vi "Dpc Get First Error.vi"(8 "error in (no error)":errorcluster, 11 "hif":u32) -> (0 "error out":errorcluster, 2 "function return":i32, 3 "hif out":u32)   [LabVIEW 2011, in "LVH-Adept.lvlib" / "DPCUTIL.lvlib"]
doc: "DPCAPI ERC DpcGetFirstError(HANDLE hif);"
uses:
  DPCUTIL.lvlib
  Resources/dpcutil.dll
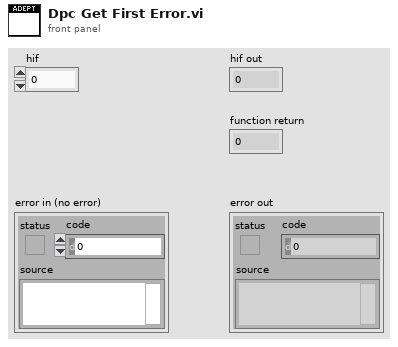
[diagram p1: front panel]
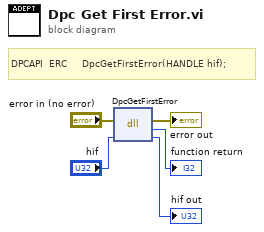
[diagram p0: block diagram]
diagram:
  # "DPCAPI  ERC     DpcGetFirstError(HANDLE hif);"
  n1 = dll-call lib="C:/github/labviewhacker/LVH-Adept/LabVIEW/vi.lib/LabVIEW Hacker/Adept/Private/Resources/dpcutil.*" fn="DpcGetFirstError"(error in="error in (no error)", "hif"="hif") -> (error out=→"error out":errorcluster, →"function return":i32, "hif"=→"hif out":u32)  [unwired: 2 in, 1 out]
